vi "Single Control Loop.vi"() -> ()   [LabVIEW 2012]
uses:
  <vilib>/Platform/TimedLoop/XDataNode/timing_clust.ctl
  <vilib>/Platform/TimedLoop/XDataNode/nitl_modes.ctl
  <vilib>/Platform/TimedLoop/XDataNode/wakeup.ctl
  <instrlib>/MicroStrain 3DM-GXx/Public/Data/Parse Message VIs/Parse (Euler Angles).vi
  <instrlib>/MicroStrain 3DM-GXx/Public/Data/Parse Message VIs/Parse (Delta Values).vi
  <instrlib>/MicroStrain 3DM-GXx/Public/Data/Parse Message VIs/Parse (Orientation Matrix).vi
  <instrlib>/MicroStrain 3DM-GXx/Public/Data/Parse Message VIs/Parse (Orientation Update Matrix).vi
  <instrlib>/MicroStrain 3DM-GXx/Public/Data/Parse Message VIs/Parse (Internal Device Temperature).vi
  <instrlib>/MicroStrain 3DM-GXx/Public/Data/Parse Message VIs/Parse (Acceleration, Angular Rate, And Magnetometer Vectors).vi
  <instrlib>/MicroStrain 3DM-GXx/Public/Data/Parse Message VIs/Parse (Gyro Stabilized Acceleration, Angular Rate, And Magnetometer Vectors).vi
  <instrlib>/MicroStrain 3DM-GXx/Public/Data/Parse Message VIs/Parse (Raw Acceleration And Angular Rates).vi
  <vilib>/platform/TimedLoop/XDataNode/XDataNode.xnode
  <instrlib>/MicroStrain 3DM-GXx/MicroStrain 3DM-GXx.lvlib
  <vilib>/Platform/TimedLoop/XDataNode/XDNodeRunTimeDep.lvlib
panel:
  in  "Reset":bool
  in  "Continuous Measurement Type":u16(ring)=5 items=["Raw Accelerometer and Angular Rate", "DeltaAngle & DeltaVelocity", "Orientation Matrix", "Orientation Update Matrix", "Acceleration, Angular Rate & Magnetometer Vectors", "Euler Angles", "Temperatures", "Gyro Stabilized Acceleration, Angular Rate & Magnetometer"]
  out "Raw Accelerometer Vector":sgl[](array[numeric])
  out "Raw Angular Rate Vector":sgl[](array[numeric])
  out "Raw Vector Timer":u32
  out "Gyro Stabilized Acceleration Vector":sgl[](array[numeric])
  out "Gyro Stabilized Angular Rate Vector":sgl[](array[numeric])
  out "Gyro Stabilized Magnetometer Vetor":sgl[](array[numeric])
  out "GS AAM Timer":u32
  out "Magnetometer Vector":sgl[](array[numeric])
  out "Acceleration 2":sgl[](array[numeric])
  out "Angular Rate 2":sgl[](array[numeric])
  out "AAM Timer":u32
  out "Magnetometer Vectors":T1(graph)
  out "Acceleration":T2(graph)
  out "Angular Rate":T3(graph)
  out "Temperature":sgl
  out "Timer":u32
  out "Orientation Update Matrix":sgl[][](array[numeric])
  out "Orientation Update Matrix Timer":u32
  out "Orientation Matrix":sgl[][](array[numeric])
  out "Orientation Matrix Timer":u32
  out "Delta Angle Vector":sgl[](array[numeric])
  out "Delta Velocity Vector":sgl[](array[numeric])
  out "Delta Timer":u32
  out "Euler Timer":u32
  out "Euler Angles":cluster{"Roll":sgl, "Pitch":sgl, "Yaw":sgl}(graph)
  out "Roll, Pitch, Yaw (Degrees)":cluster{dbl, dbl, dbl}(knob) caption="Red Green Blue" scale=-180.0..180.0
  in  "Stop":bool
  in  "VISA resource name":refnum<visa-resource-name>="ASRL1::INSTR"
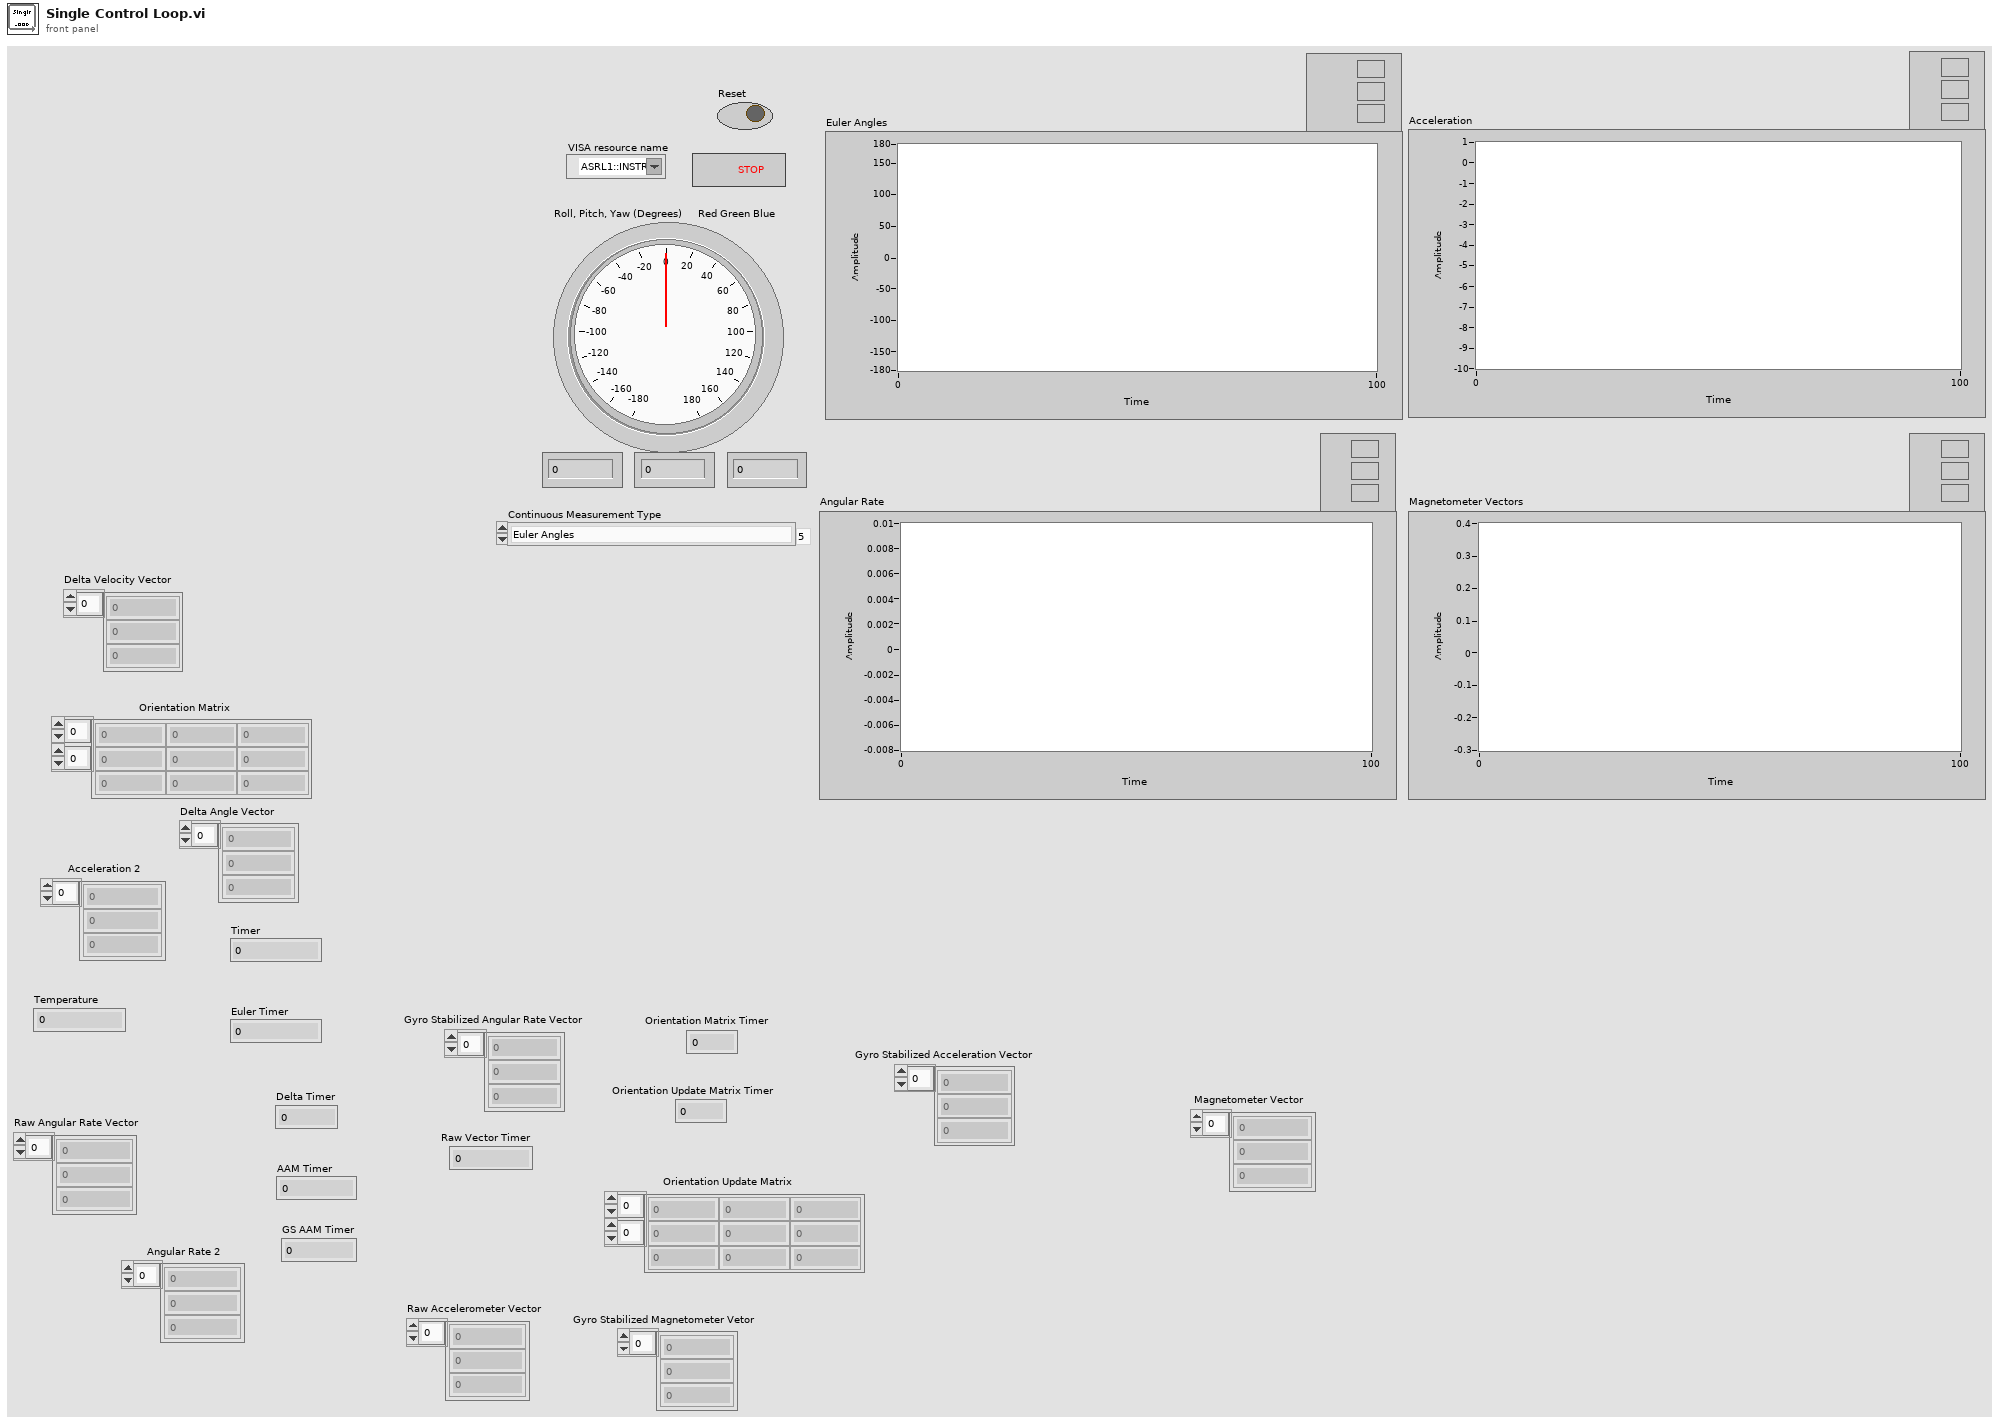
[diagram p1: front panel]
types:
  T1 = cluster{"Magnetometer Vector[0]":sgl, "Magnetometer Vector[1]":sgl, "Magnetometer Vector[2]":sgl, "Magnetometer Vector[3]":sgl, "Magnetometer Vector[4]":sgl, "Magnetometer Vector[5]":sgl, "Magnetometer Vector[6]":sgl, "Magnetometer Vector[7]":sgl, "Magnetometer Vector[8]":sgl}
  T2 = cluster{"Acceleration[0]":sgl, "Acceleration[1]":sgl, "Acceleration[2]":sgl, "Acceleration[3]":sgl, "Acceleration[4]":sgl, "Acceleration[5]":sgl, "Acceleration[6]":sgl, "Acceleration[7]":sgl, "Acceleration[8]":sgl}
  T3 = cluster{"Angular Rate[0]":sgl, "Angular Rate[1]":sgl, "Angular Rate[2]":sgl, "Angular Rate[3]":sgl, "Angular Rate[4]":sgl, "Angular Rate[5]":sgl, "Angular Rate[6]":sgl, "Angular Rate[7]":sgl, "Angular Rate[8]":sgl}
  T4 = typedef "XDNodeRunTimeDep.lvlib/timing_clust.ctl" = cluster{"Expected End [f-1]":u64, "Actual End [f-1]":u64, "Finished Late? [f-1]":bool, "Expected End [i-1]":u64, "Actual End [i-1]":u64, "Finished Late? [i-1]":bool, "Expected Start [i]":u64, "Actual Start [i]":u64, "Expected Start [f]":u64, "Actual Start [f]":u64, "Source Name":string, "Structure Name":string, "Period":i64, "Deadline":i64, "Offset":i64, "Start":i64, "Priority":i32, "Timeout":i32, "Mode":T5, "Wakeup Reason":T6, "Error":errorcluster, "Source Type":string, "Secondary Source Type":string, "Global End Time":u64, "Global Start Time":u64, "Frame Duration":u64, "Iteration Duration":u64, "Assigned CPU":i32, "I/O Scan Engine Mode":u32}
  T5 = typedef "XDNodeRunTimeDep.lvlib/nitl_modes.ctl" = enum32{"No Change", "Process missed periods, maintain original phase", "Discard missed periods, maintain original phase", "Process missed periods, ignore original phase", "Discard missed periods, ignore original phase"}
  T6 = typedef "XDNodeRunTimeDep.lvlib/wakeup.ctl" = enum32{"Normal", "Aborted", "Asynchronous wakeup", "Timing source error", "Timed loop error", "Timeout"}
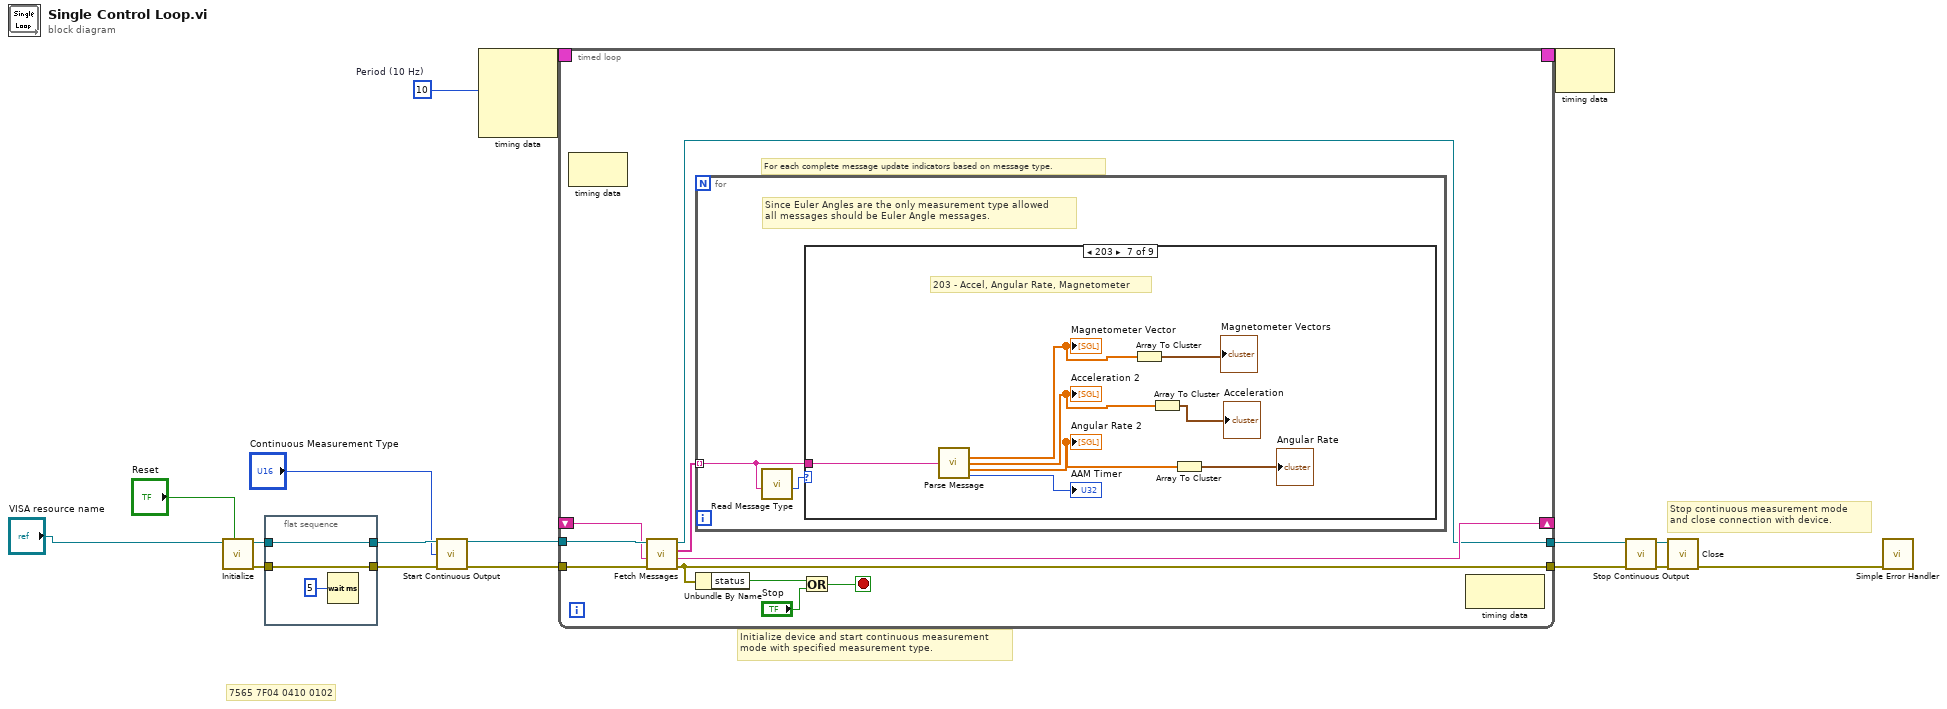
[diagram p0: block diagram]
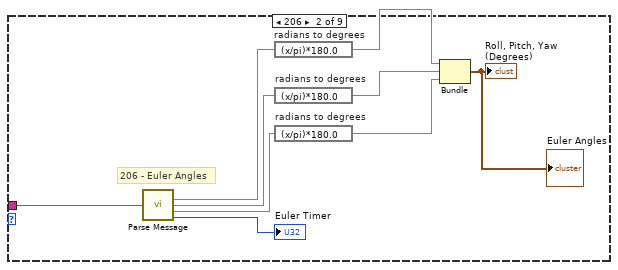
[diagram p3: hidden frame]
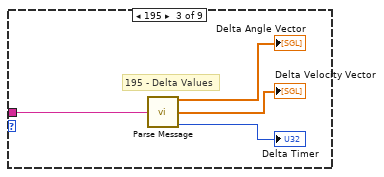
[diagram p4: hidden frame]
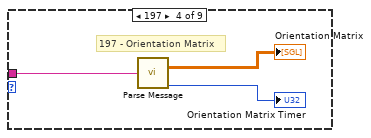
[diagram p5: hidden frame]
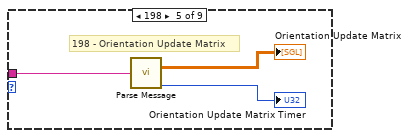
[diagram p6: hidden frame]
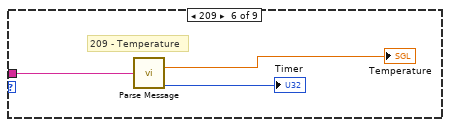
[diagram p7: hidden frame]
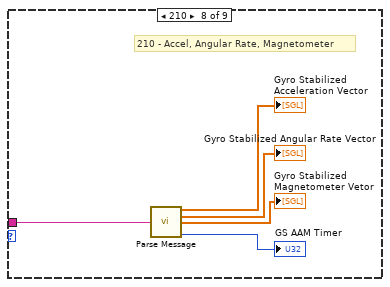
[diagram p8: hidden frame]
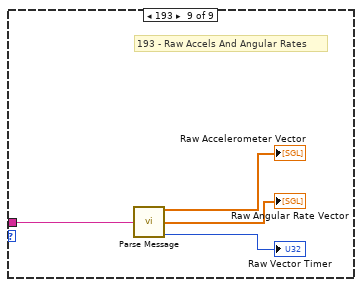
[diagram p9: hidden frame]
diagram:
  w1 = i64 10  # Period (10 Hz)
  # "7565 7F04 0410 0102"
  # "Stop continuous measurement mode \nand close connection with device."
  # "Initialize device and start continuous measurement \nmode with specified measurement type."
  n1 = call <instrlib>:"Initialize.vi"("Reset (False)"="Reset", "VISA resource name"="VISA resource name") -> ("error out"=w7:errorcluster, "VISA resource name out"=w5:refnum<visa-resource-name>)  [unwired: 8 in]
  n2 = flat-sequence {
    tunnel: [w19] -> w8
    tunnel: w7 -> [w19]
    tunnel: [w18] -> w6
    tunnel: w5 -> [w18]
    frame #0 {
      n3 = Wait (ms)(milliseconds to wait=u32 5) -> ()  [unwired: 1 out]
    }
  }
  n4 = call <instrlib>:"Start Continuous Output.vi"("VISA resource name"=w6, "Continuous Measurement Type (Raw Accelerometer and Angular Rate)"="Continuous Measurement Type", "error in (no error)"=w8) -> ("VISA resource name out"=w15:refnum<visa-resource-name>, "error out"=w14:errorcluster)  [unwired: 11 in]
  n5 = node-c288(w1) -> (w17:T4)  [unwired: 3 in]
  n6 = timed-loop {
    tunnel: w15 -> [w30]
    tunnel: w14 -> [w29]
    shift-right: [w27] -> _
    shift-left: _ -> [w28]
    tunnel: [w25] -> w13
    tunnel: [w24] -> w12
    timing: w17 -> [_]
    timing-out: [_] -> w16
    stop <- w21 stop-if-true
    # "For each complete message update indicators based on message type."
    n7 = node-c288() -> ()  [unwired: 1 in, 1 out]
    n8 = call <instrlib>:"Fetch Messages.vi"("error in (no error)"=w29, "Remainder In"=w28, "VISA resource name"=w30) -> ("error out"=w24:errorcluster, "Remainder Out"=w27:string, "Complete Messages"=w26:string[], "VISA resource name out"=w25:refnum<visa-resource-name>)  [unwired: 5 in]
    n9 = for {
      tunnel: w26 -> [w34] mode=indexing
      # "Since Euler Angles are the only measurement type allowed \nall messages should be Euler Angle messages."
      n10 = call <instrlib>:"Read Message Type.vi"("Message"=w34) -> ("Ring"=w33:u16)  [unwired: 10 in]
      n11 = case shown="203" w33 {
        tunnel: w34 -> [_ w43 w47 w50 w53 w56 w64 w69 w73]
        frame 0, Default {
          # "Unknown message type. \nDisregard message."
        }
        frame 206 {
          # "206 - Euler Angles"
          n12 = call-poly <instrlib>:"Parse Message.vi"("Message In"=w43) -> ("Roll"=w41:sgl, "Pitch"=w40:sgl, "Yaw"=w39:sgl, "Timer"=→"Euler Timer":u32)  [unwired: 11 in]
          n13 = expression code="(x/pi)*180.0" "radians to degrees"(w41) -> (w38:sgl)
          n14 = expression code="(x/pi)*180.0" "radians to degrees"(w40) -> (w37:sgl)
          n15 = expression code="(x/pi)*180.0" "radians to degrees"(w39) -> (w36:sgl)
          n16 = Bundle("Roll"=w38, "Pitch"=w37, "Yaw"=w36) -> (→"Euler Angles" →"Roll, Pitch, Yaw (Degrees)":cluster{"Roll":sgl, "Pitch":sgl, "Yaw":sgl})  [unwired: 1 in]
        }
        frame 195 {
          # "195 - Delta Values"
          n17 = call-poly <instrlib>:"Parse Message.vi"("Message In"=w47) -> ("DeltaAngleVector"=→"Delta Angle Vector":sgl[], "DeltaVelocityVector"=→"Delta Velocity Vector":sgl[], "Timer"=→"Delta Timer":u32)  [unwired: 12 in]
        }
        frame 197 {
          # "197 - Orientation Matrix"
          n18 = call-poly <instrlib>:"Parse Message.vi"("Message In"=w50) -> ("Orientation Matrix"=→"Orientation Matrix":sgl[][], "Timer"=→"Orientation Matrix Timer":u32)  [unwired: 13 in]
        }
        frame 198 {
          # "198 - Orientation Update Matrix"
          n19 = call-poly <instrlib>:"Parse Message.vi"("Message In"=w53) -> ("Orientation Update Matrix"=→"Orientation Update Matrix":sgl[][], "Timer"=→"Orientation Update Matrix Timer":u32)  [unwired: 13 in]
        }
        frame 209 {
          # "209 - Temperature"
          n20 = call-poly <instrlib>:"Parse Message.vi"("Message In"=w56) -> ("Temperature"=→"Temperature":sgl, "Timer"=→"Timer":u32)  [unwired: 13 in]
        }
        frame 203 {
          # "203 - Accel, Angular Rate, Magnetometer"
          n21 = call-poly <instrlib>:"Parse Message.vi"("Message In"=w64) -> ("Magnetometer Vector"=w62:sgl[], "Acceleration"=w60:sgl[], "Angular Rate"=w58:sgl[], "Timer"=→"AAM Timer":u32)  [unwired: 11 in]
          "Magnetometer Vector" <- w62
          "Acceleration 2" <- w60
          "Angular Rate 2" <- w58
          n22 = Array To Cluster(array=w62) -> (cluster=→"Magnetometer Vectors":T1)
          n23 = Array To Cluster(array=w60) -> (cluster=→"Acceleration":T2)
          n24 = Array To Cluster(array=w58) -> (cluster=→"Angular Rate":T3)
        }
        frame 210 {
          # "210 - Accel, Angular Rate, Magnetometer"
          n25 = call-poly <instrlib>:"Parse Message.vi"("Message In"=w69) -> ("Gyro Stabilized Acceleration Vector"=→"Gyro Stabilized Acceleration Vector":sgl[], "Gyro Stabilized Angular Rate Vector"=→"Gyro Stabilized Angular Rate Vector":sgl[], "Gyro Stabilized Magnetometer Vetor"=→"Gyro Stabilized Magnetometer Vetor":sgl[], "Timer"=→"GS AAM Timer":u32)  [unwired: 11 in]
        }
        frame 193 {
          # "193 - Raw Accels And Angular Rates"
          n26 = call-poly <instrlib>:"Parse Message.vi"("Message In"=w73) -> ("Raw Accelerometer Vector"=→"Raw Accelerometer Vector":sgl[], "Raw Angular Rate Vector"=→"Raw Angular Rate Vector":sgl[], "Timer"=→"Raw Vector Timer":u32)  [unwired: 12 in]
        }
      }
    }
    n27 = Unbundle By Name(w24) -> ("status"=w23:bool)
    n28 = Or(x=w23, y="Stop") -> (x .or. y?=w21:bool)
    n29 = node-c288() -> ()  [unwired: 1 in, 1 out]
  }
  n30 = node-c288(w16) -> ()  [unwired: 1 out]
  n31 = call <instrlib>:"Stop Continuous Output.vi"("error in (no error)"=w12, "VISA resource name"=w13) -> ("error out"=w11:errorcluster, "VISA resource name out"=w10:refnum<visa-resource-name>)  [unwired: 8 in]
  n32 = call <instrlib>:"Close.vi"("error in (no error)"=w11, "VISA resource name"=w10) -> ("error out"=w9:errorcluster)  [unwired: 9 in]
  n33 = call <vilib>:"Simple Error Handler.vi"("error in (no error)"=w9) -> ()  [unwired: 4 in, 5 out]
